vi "Command Type.vi"(11 "Command in":refnum<class "Command.lvclass">) -> (2 "Command Type":string)   [LabVIEW 2020, in "VolatusSeq.lvlib" / "Command.lvclass"]
uses:
  Command.lvclass
  Command.lvclass/Command.ctl
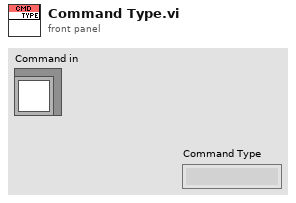
[diagram p1: front panel]
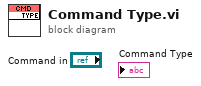
[diagram p0: block diagram]
diagram:
